vi "Add MyTopic Writer Channels.vi"(8 "error in (no error)":errorcluster, 11 "nodeID":u64) -> (0 "error out":errorcluster, 3 "nodeID out":u64)   [LabVIEW 2015, in "DDS Custom Device System Explorer.lvlib"]
uses:
  DDS Custom Device System Explorer.lvlib
  <vilib>/NI Veristand/Custom Device API/Custom Device Channel.ctl
  <vilib>/NI Veristand/Custom Device API/Custom Device Channel Type.ctl
  Shared/Constants.vi
  <vilib>/ni/NI VeriStand Advanced SysDef API/SysDef API/Advanced System Definition.lvlib
  Shared/DDS Custom Device Shared.lvlib
  <vilib>/NI VeriStand/Custom Device API/Custom Device API.lvlib
  <vilib>/NI VeriStand/Custom Device Tools/Custom Device Utility Library/Custom Device Utility Library.lvlib
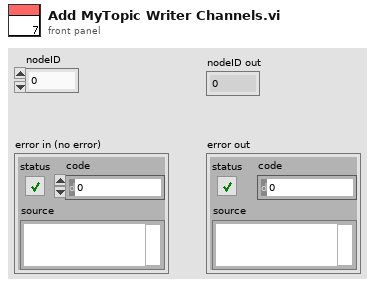
[diagram p1: front panel]
types:
  T1 = typedef "Custom Device API.lvlib/Custom Device Channel.ctl" = cluster{"Type":T2, "Units":string, "Default Value":dbl, "Faultable":bool, "Scalable":bool}
  T2 = typedef "Custom Device API.lvlib/Custom Device Channel Type.ctl" = enum16{"Input", "Output"}
  T3 = typedef "Custom Device API.lvlib/Custom Device Item Ref.ctl" = u64
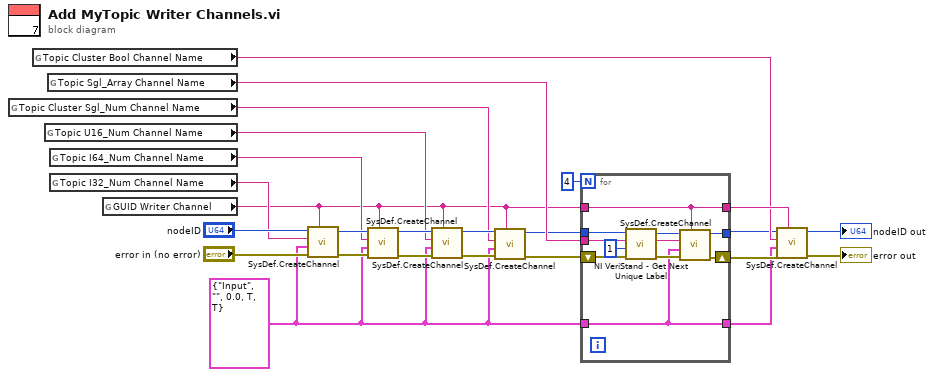
[diagram p0: block diagram]
diagram:
  w9 = T1 {"Type"=enum."Input", "Units"="", "Default Value"=0.0, "Faultable"=TRUE, "Scalable"=TRUE} ("Channel")
  n1 = global read "Constants.vi" "Topic Cluster Sgl_Num Channel Name"() -> (w14:string)
  n2 = global read "Constants.vi" "Topic Cluster Bool Channel Name"() -> (w5:string)
  n3 = global read "Constants.vi" "Topic U16_Num Channel Name"() -> (w17:string)
  n4 = global read "Constants.vi" "Topic Sgl_Array Channel Name"() -> (w12:string)
  n5 = global read "Constants.vi" "Topic I64_Num Channel Name"() -> (w20:string)
  n6 = global read "Constants.vi" "Topic I32_Num Channel Name"() -> (w23:string)
  n7 = global read "Constants.vi" "GUID Writer Channel"() -> (w8:string)
  n8 = call <vilib>:"SysDef.CreateChannel.vi"("GUID"=w8, "error in (no error)"="error in (no error)", "Channel"=w9, "Name"=w23, "nodeID"="nodeID") -> ("error out"=w22:errorcluster, "nodeID out"=w21:u64)  [unwired: 3 in, 2 out]
  n9 = call <vilib>:"SysDef.CreateChannel.vi"("GUID"=w8, "error in (no error)"=w22, "Channel"=w9, "Name"=w20, "nodeID"=w21) -> ("error out"=w18:errorcluster, "nodeID out"=w19:u64)  [unwired: 3 in, 2 out]
  n10 = call <vilib>:"SysDef.CreateChannel.vi"("GUID"=w8, "error in (no error)"=w18, "Channel"=w9, "Name"=w17, "nodeID"=w19) -> ("error out"=w15:errorcluster, "nodeID out"=w16:u64)  [unwired: 3 in, 2 out]
  n11 = call <vilib>:"SysDef.CreateChannel.vi"("GUID"=w8, "error in (no error)"=w15, "Channel"=w9, "Name"=w14, "nodeID"=w16) -> ("error out"=w13:errorcluster, "nodeID out"=w10:u64)  [unwired: 3 in, 2 out]
  n12 = for {
    N: 4 -> [_]
    tunnel: w12 -> [w35]
    tunnel: w10 -> [w34]
    tunnel: w9 -> [w26]
    tunnel: w8 -> [w27]
    shift-right: [w29] -> w7
    shift-left: w13 -> [w36]
    tunnel: [w28] -> w3
    tunnel: [w27] -> w6
    tunnel: [w26] -> w4
    n13 = call <vilib>:"NI VeriStand - Get Next Unique Label.vi"("error in (no error)"=w36, "Start Value (1)"=1, "Label"=w35, "Parent Ref in"=w34) -> ("error out"=w32:errorcluster, "Label out"=w31:string, "Parent Ref dup"=w30:T3)  [unwired: 4 in, 1 out]
    n14 = call <vilib>:"SysDef.CreateChannel.vi"("GUID"=w27, "error in (no error)"=w32, "Channel"=w26, "Name"=w31, "nodeID"=w30) -> ("error out"=w29:errorcluster, "nodeID out"=w28:u64)  [unwired: 3 in, 2 out]
  }
  n15 = call <vilib>:"SysDef.CreateChannel.vi"("GUID"=w6, "error in (no error)"=w7, "Channel"=w4, "Name"=w5, "nodeID"=w3) -> ("error out"=→"error out":errorcluster, "nodeID out"=→"nodeID out":u64)  [unwired: 3 in, 2 out]
